vi "Main.vi"(11 "Module Admin":refnum<class "Delacor_lib_QMH_Module Admin.lvclass">) -> ()   [LabVIEW 2020, in "Graficas.lvlib"]
doc: "This template is based off of the Queued Message Handler design pattern and the Queued Message Handler project template that ships with LabVIEW.\n\nThe main difference is that the queue is private to this module and communication between modules is performed via Broadcast and Request events.\n\nRequest events are wrapped in public API methods and are handled in the Event Handling Loop (EHL) of this VI. Any module can register for Broadcast events sent by this module. The EHL generates messages based on user interface actions.\n\nThe Message Handling Loop (MHL) processes messages generated by the EHL, or by other messages. The messages are string values, so new messages can be added easily to the Message Cases case structure in the MHL. Each message cluster can also provide an optional value for Message Data, which is a variant that can be converted to whatever message-specific data is required.\n_____\nBased on Delacor QMH Project Template 5.0.0.82."
uses:
  Graficas.lvlib
  <vilib>/Delacor/Delacor QMH/Libraries/Module Admin_class/Delacor_lib_QMH_Module Admin.lvclass
  Module Data--cluster.ctl
  <vilib>/Delacor/Delacor QMH/Libraries/Message Queue_class/Delacor_lib_QMH_Message Queue.lvclass/Delacor_lib_QMH_Message Queue.ctl
  Stop Argument--cluster.ctl
  <vilib>/Delacor/Delacor QMH/Libraries/Module Admin_class/Delacor_lib_QMH_Module Admin.lvclass/Delacor_lib_QMH_Module Admin.ctl
  Mostrar en SubPanel Argument--cluster.ctl
  <vilib>/Utility/miscctls.llb/LVPointTypeDef.ctl
  <vilib>/Delacor/Delacor QMH/Libraries/Message Queue_class/Delacor_lib_QMH_Enqueue Message (Single).vi
  <vilib>/Delacor/Delacor QMH/Libraries/Module Admin_class/Delacor_lib_QMH_Get External Launch.vi
  <vilib>/Utility/error.llb/Error Cluster From Error Code.vi
  <vilib>/ErrorRing/Error Ring.xnode
  <vilib>/Delacor/Delacor QMH/Libraries/Message Queue_class/Delacor_lib_QMH_Message Queue.lvclass
  Main/Main.lvlib
panel:
  out "Grafica Excitacion":dbl(graph)
  out "Grafica Voltajes":T1(graph)
  out "Grafica SOC":dbl(graph)
  out "Grafica Corriente":dbl(graph)
  out "SOC de Batería":dbl=80.0 format="%_5f %%"
  out "Voltaje de Batería":dbl=270.0 format="%.1f V"
  out "Corriente Excitación":dbl=2.0 format="%_3f A"
  out "Potencia Generador":dbl=300.0 format="%.1f kW"
  out "Corriente Generador":dbl=1000.0 format="%.1f A"
  out "Voltaje Generador":dbl=288.0 format="%.1f V"
  out "error out":errorcluster
  out "Status":string
  # "Tendencias del Generador"
  # "Voltaje Generador / Batería"
  # "Corriente del Generador"
  # "Indicadores Generador"
  # "Estado de Carga de Batería"
  # "Corriente de Excitación"
  # "Indicadores Batería"
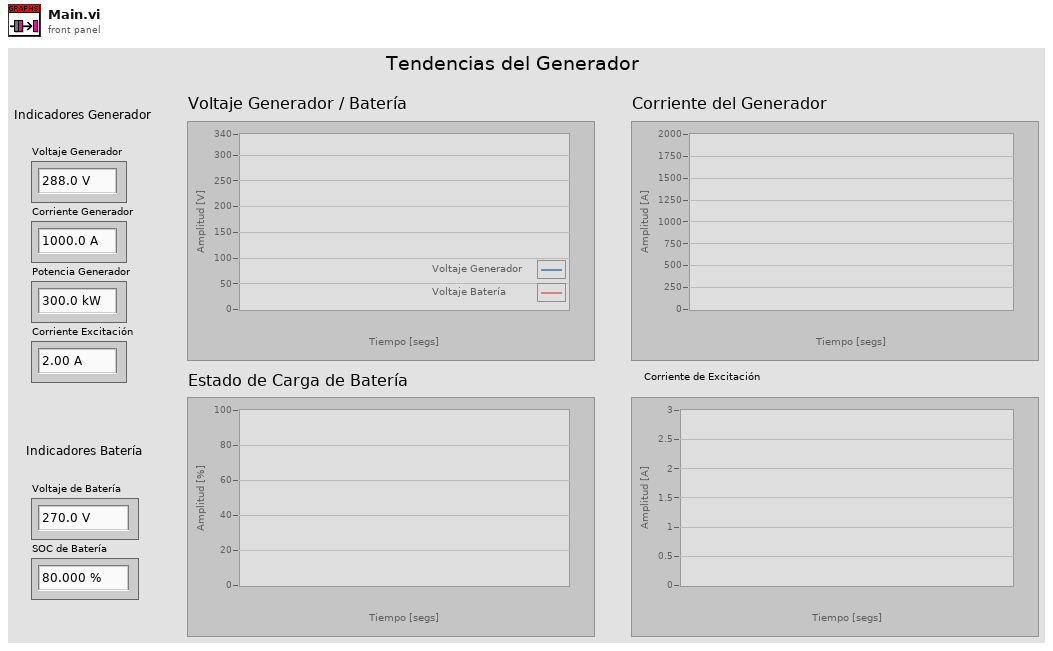
[diagram p1: front panel]
types:
  T1 = cluster{"Voltaje Generador":dbl, "Voltaje de Batería":dbl}
  T2 = typedef "Graficas.lvlib/Request Events--cluster.ctl" = cluster{"Stop Module":refnum<user-event>, "Show Panel":refnum<user-event>, "Hide Panel":refnum<user-event>, "Get Module Execution Status":refnum<user-event>, "Show Diagram":refnum<user-event>, "Mostrar en SubPanel":refnum<user-event>}
  T3 = typedef "Main.lvlib/Broadcast Events--cluster.ctl" = cluster{"Module Did Init":refnum<user-event>, "Status Updated":refnum<user-event>, "Error Reported":refnum<user-event>, "Module Did Stop":refnum<user-event>, "Update Module Execution Status":refnum<user-event>, "Generador Encendido-Apagado":refnum<user-event>}
  T4 = typedef "Graficas.lvlib/Module Data--cluster.ctl" = cluster{"Status":string}
  T5 = enum32{"invalid lock state", "Not Locked", "Locked (No Password)", "Password-protected"}
  T6 = typedef "Graficas.lvlib/Stop Argument--cluster.ctl" = cluster{"Origin":string, "Exit via Stop Module Req?":bool, "Wait for Module to stop?":bool}
  T7 = typedef "Graficas.lvlib/Mostrar en SubPanel Argument--cluster.ctl" = cluster{"SubPnl Refnum":refnum<vi>}
  T8 = cluster{"current time":timestamp, "Voltaje Generador":dbl, dbl}[]
  T9 = typedef "LVPointTypeDef.ctl" = cluster{"Horizontal":i16, "Vertical":i16}
  T10 = enum32{"Invalid", "Standard", "Closed", "Hidden", "Minimized", "Maximized"}
  T11 = cluster{"Voltaje Generador":dbl, "Voltaje de Batería":dbl}[]
  T12 = cluster{"current time":timestamp, "Corriente Generador":dbl}[]
  T13 = enum8{"Enabled", "Disabled", "Disabled and Grayed Out"}
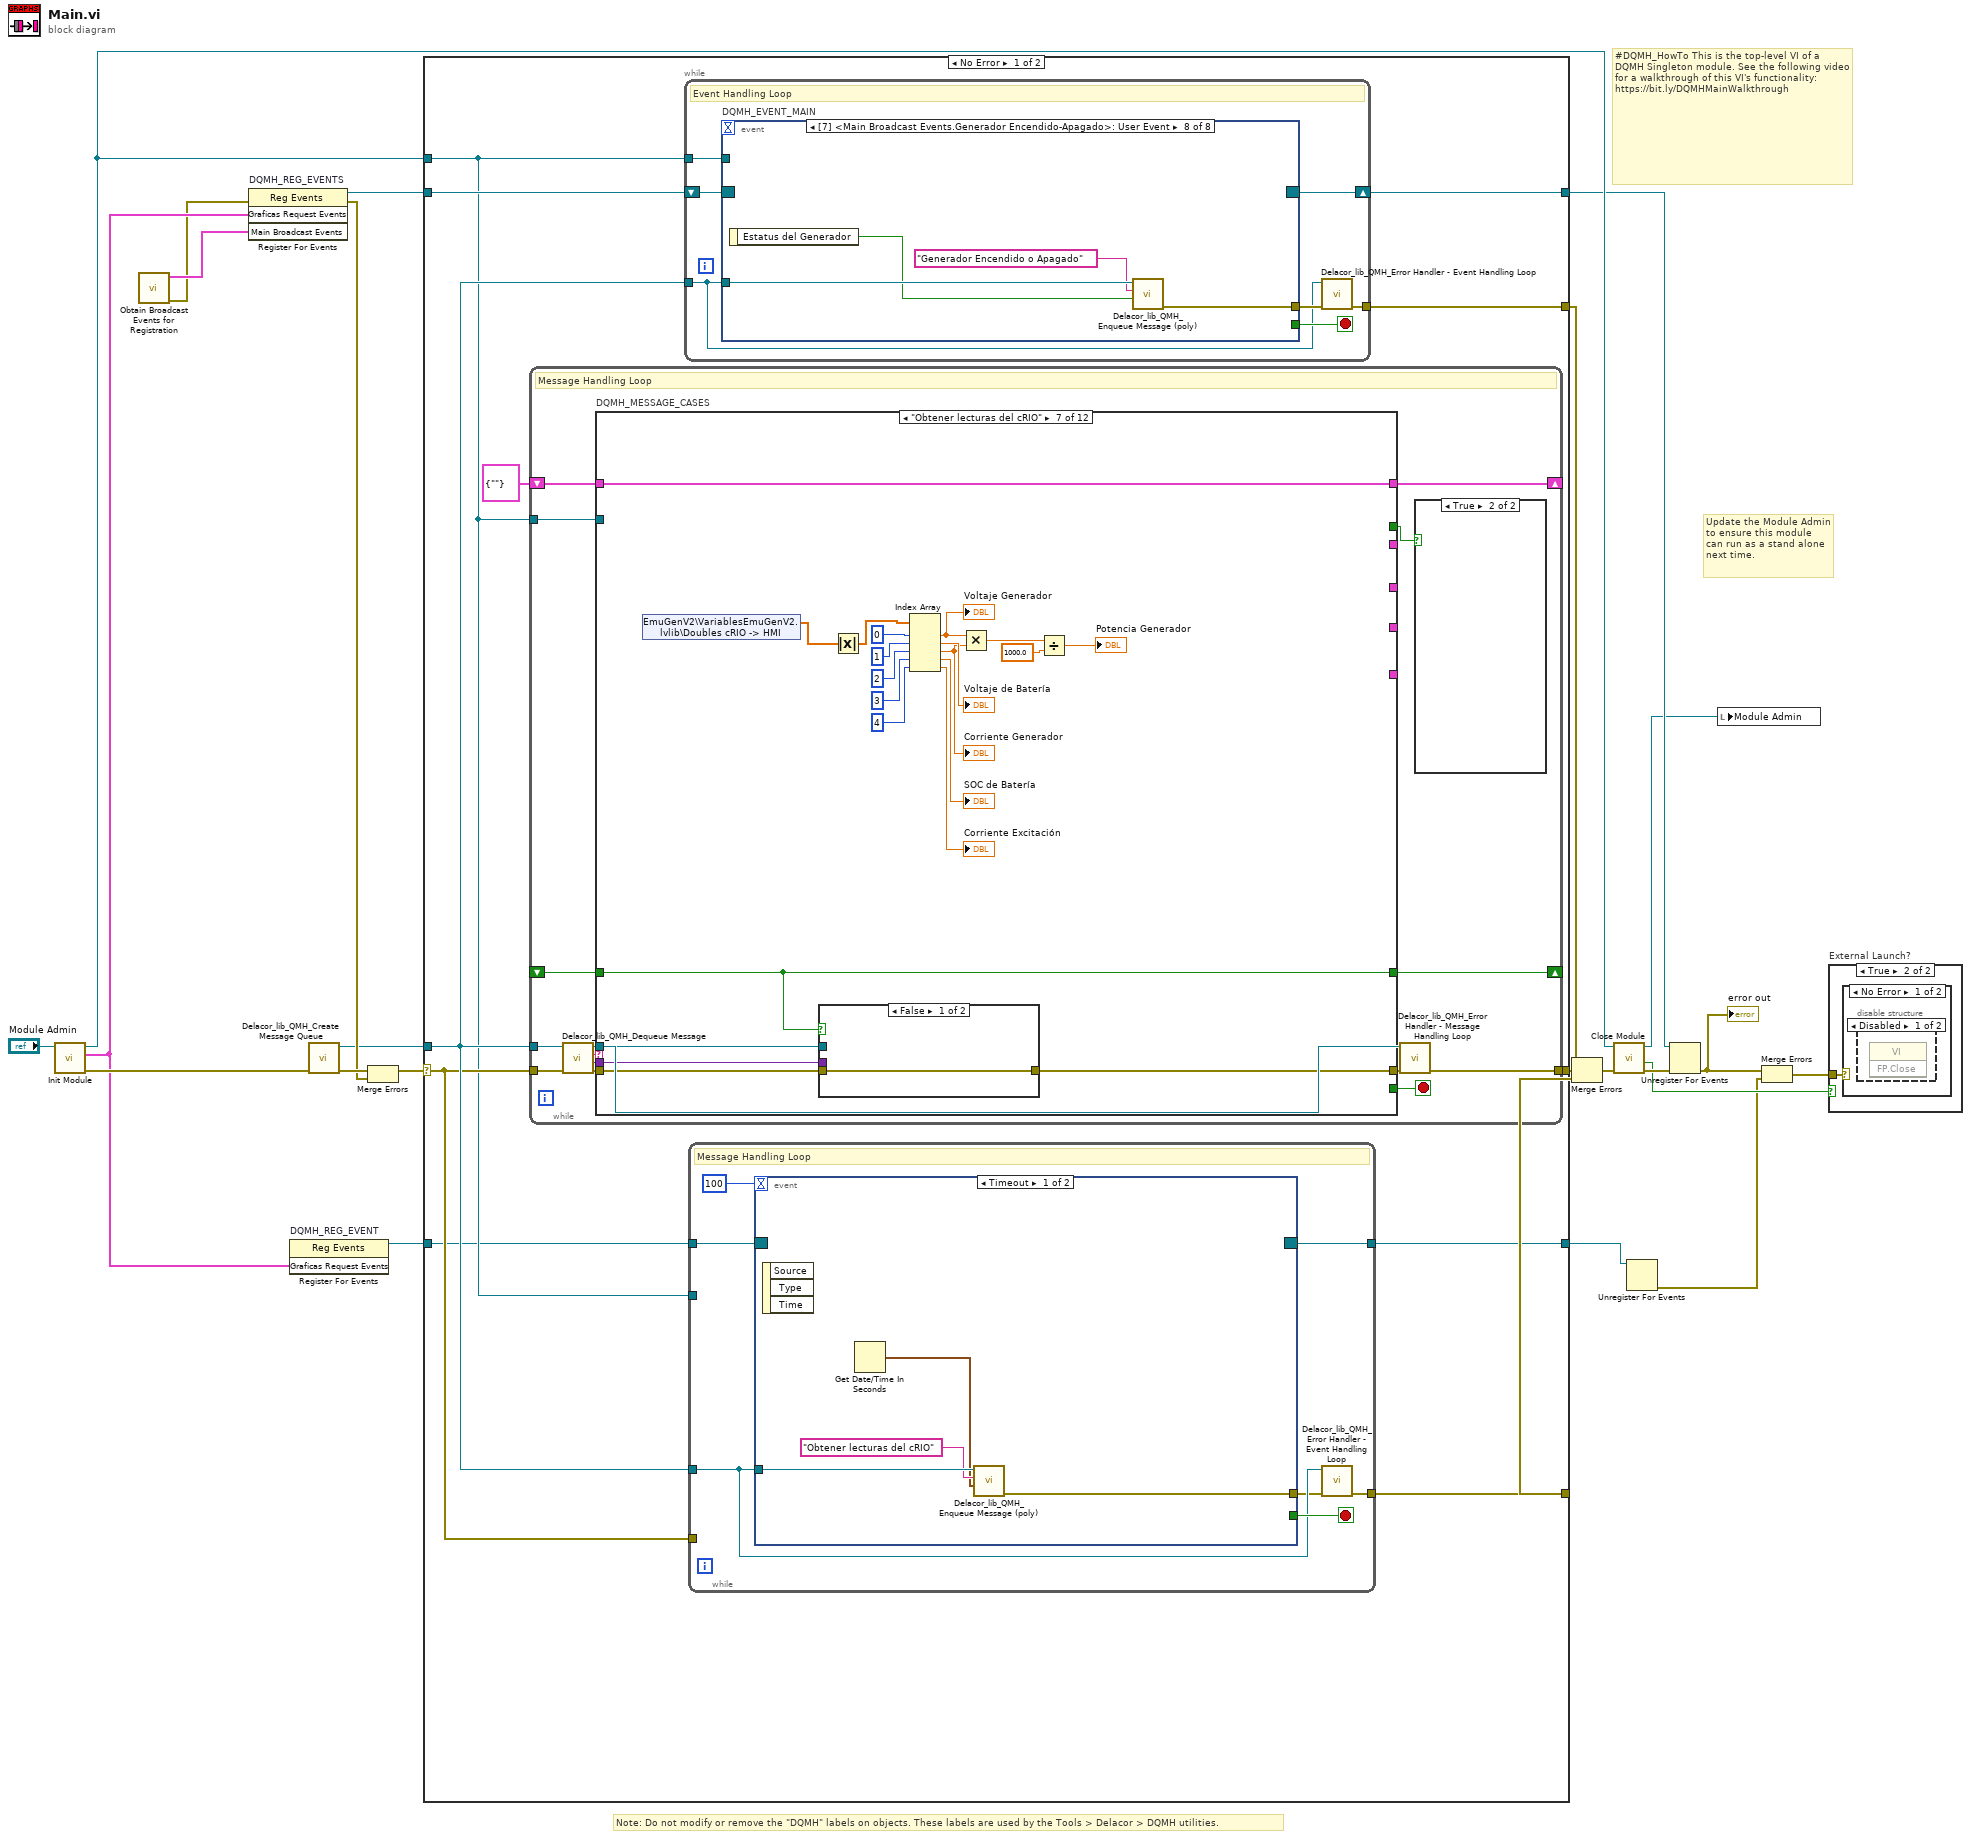
[diagram p0: block diagram]
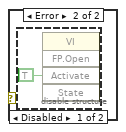
[diagram p4: hidden frame]
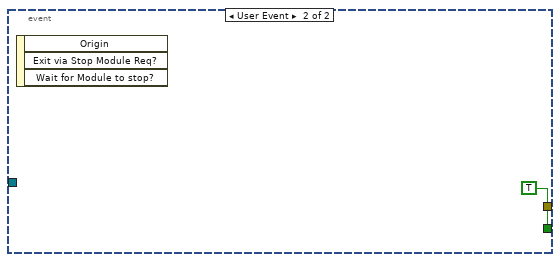
[diagram p6: hidden frame]
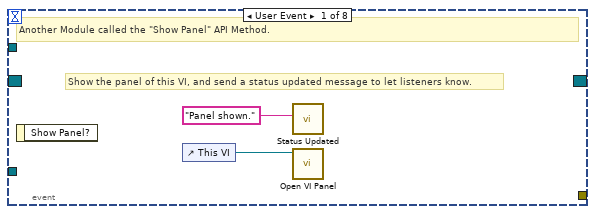
[diagram p7: hidden frame]
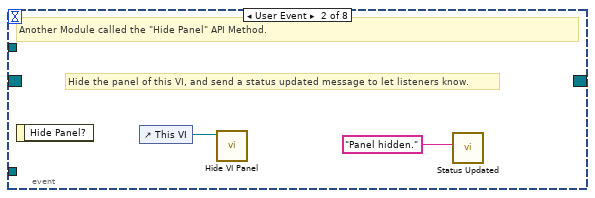
[diagram p8: hidden frame]
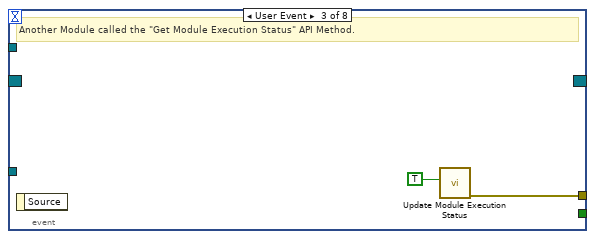
[diagram p9: hidden frame]
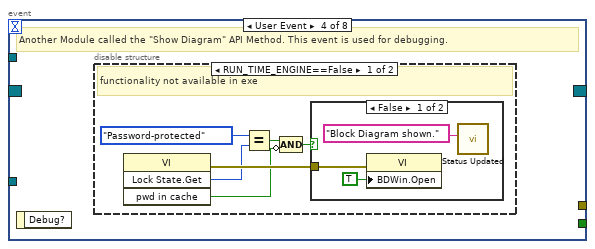
[diagram p10: hidden frame]
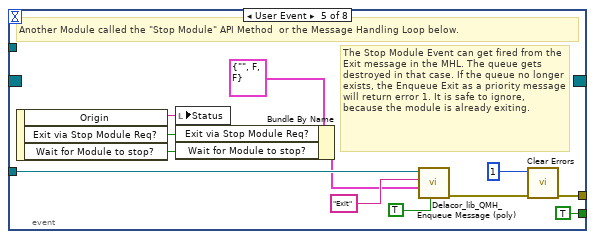
[diagram p13: hidden frame]
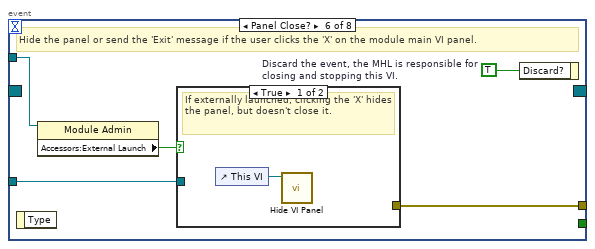
[diagram p14: hidden frame]
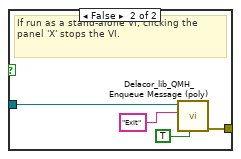
[diagram p15: hidden frame]
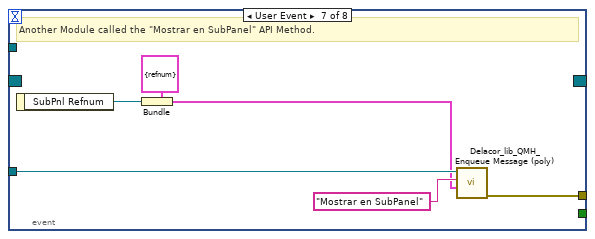
[diagram p16: hidden frame]
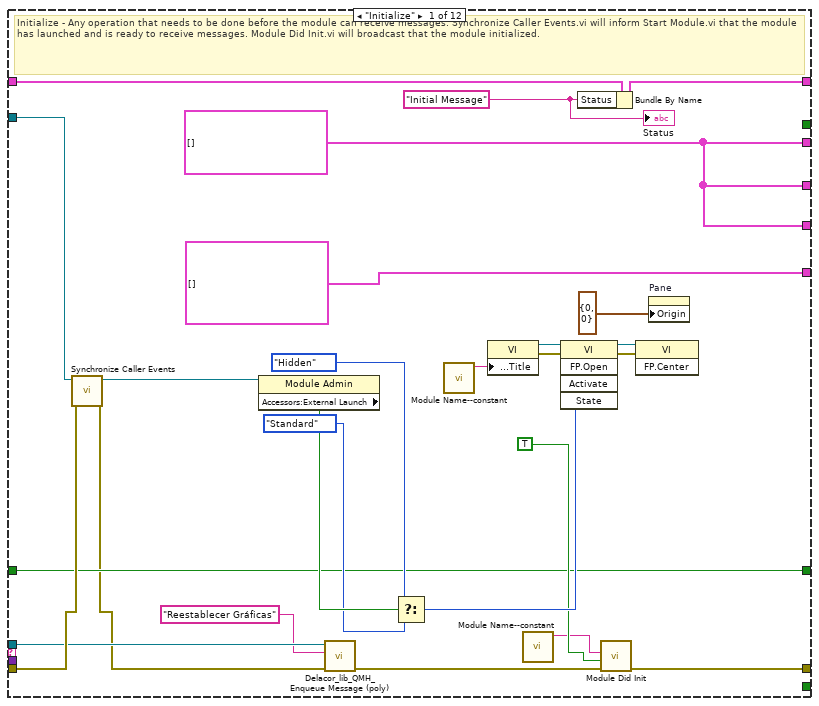
[diagram p18: hidden frame]
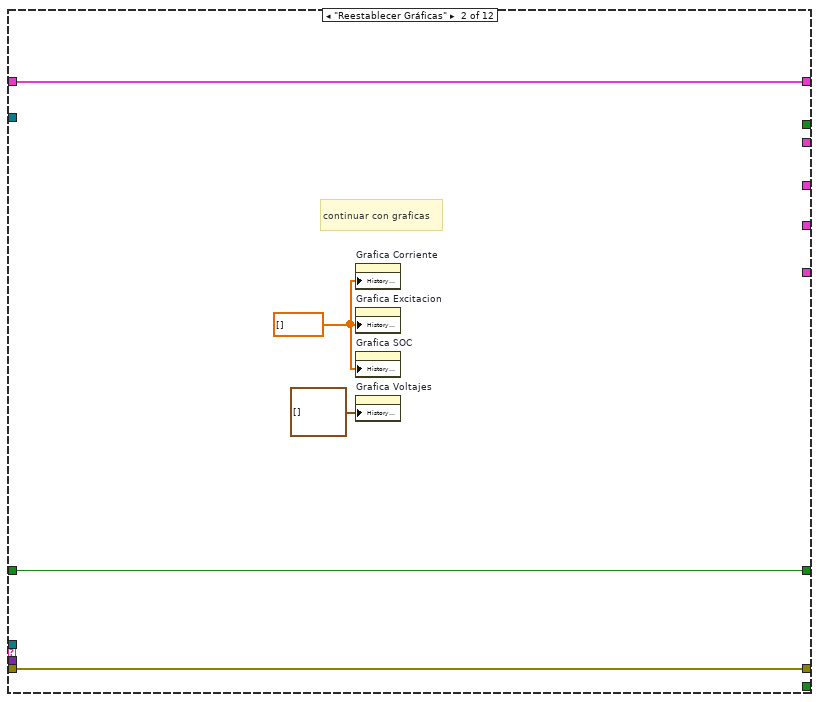
[diagram p19: hidden frame]
diagram:
  # "#DQMH_HowTo This is the top-level VI of a DQMH Singleton module. See the following video for a walkthrough of this VI's functionality: https://bit.ly/DQMHMainWalkthrough"
  # "Note: Do not modify or remove the \"DQMH\" labels on objects. These labels are used by the Tools > Delacor > DQMH utilities."
  # "Update the Module Admin to ensure this module can run as a stand alone next time."
  n1 = call "Init Module.vi"("Singleton Module Admin in"="Module Admin") -> ("error out"=w23:errorcluster, "Graficas Request Events"=w9:T2, "Singleton Module Admin out"=w16:refnum<class "Delacor_lib_QMH_Module Admin.lvclass">)  [unwired: 8 in]
  n2 = call "Obtain Broadcast Events for Registration.vi"() -> ("error out"=w1:errorcluster, "Main Broadcast Events"=w2:T3)  [unwired: 9 in, 1 out]
  n3 = register-events "DQMH_REG_EVENTS"(error in=w1, w9, w2) -> (reference out=w14:refnum<event-registration>, error out=w17:errorcluster)  [unwired: 1 in]
  n4 = register-events "DQMH_REG_EVENT"(w9) -> (reference out=w8:refnum<event-registration>)  [unwired: 2 in, 1 out]
  n5 = call <vilib>:"Delacor_lib_QMH_Create Message Queue.vi"("error in (no error)"=w23) -> ("error out"=w19:errorcluster, "Message Queue"=w13:refnum<class "Delacor_lib_QMH_Message Queue.lvclass">)  [unwired: 9 in]
  n6 = Merge Errors(w19, w17) -> (w18:errorcluster)
  n7 = case shown="No Error" w18 {
    selector: w18 -> [w29 w274]
    tunnel: [w35 w273] -> w24
    tunnel: [w33 w279] -> w15
    tunnel: w14 -> [w31 w279]
    tunnel: w13 -> [w30 w272]
    tunnel: [w34 _] -> w21
    tunnel: w16 -> [w28 w275]
    tunnel: w8 -> [w27 w271]
    tunnel: [w26 w271] -> w7
    tunnel: [w25 _] -> w3
    frame No Error {
      n8 = while {
        tunnel: w30 -> [w107]
        shift-right: [w111] -> _
        shift-left: T4 {"Status"=""} ("Data Cluster") -> [w112]
        tunnel: w29 -> [w115]
        tunnel: [w113] -> w35
        tunnel: w28 -> [w105]
        shift-right: [w103] -> _
        shift-left: _ -> [w102]
        stop <- w110 stop-if-true
        # "Message Handling Loop"
        n9 = call-dynamic "Delacor_lib_QMH_Dequeue Message.vi"("error in (no error)"=w115, "Message Queue in"=w107) -> ("error out"=w114:errorcluster, "Message Data"=w108:variant, "Message"=w109:string, "Message Queue out"=w106:refnum<class "Delacor_lib_QMH_Message Queue.lvclass">)  [unwired: 6 in]
        n10 = case "DQMH_MESSAGE_CASES" shown="\"Obtener lecturas del cRIO\"" w109 {
          selector: w109 -> [_ _ _ _ _ _ _ _ _ _ _ w258]
          tunnel: w106 -> [w120 _ _ _ _ w167 w200 _ _ w226 w249 _]
          tunnel: w114 -> [w140 w147 w150 w160 w164 w171 w199 w218 w221 w233 w255 w260]
          tunnel: [w139 w147 w150 w152 w163 w173 w198 w217 w221 w229 w252 w261] -> w116
          tunnel: w112 -> [w130 w146 w149 w159 w162 w172 w201 w216 w220 w228 w248 w259]
          tunnel: [w129 w146 w149 w159 w162 w172 w201 w216 w220 w228 w248 w259] -> w111
          tunnel: [_ _ _ _ _ _ _ _ _ _ w247 _] -> w110
          tunnel: w108 -> [_ _ _ w158 _ w170 w197 _ _ w227 w246 _]
          tunnel: w105 -> [w131 _ _ _ _ _ _ _ _ w225 w241 _]
          tunnel: [T8 [] _ _ _ _ _ _ _ _ _ _ _] -> _
          tunnel: [w122 _ _ _ _ _ _ _ _ _ _ _] -> _
          tunnel: [w122 _ _ _ _ _ _ _ _ _ _ _] -> _
          tunnel: [w122 _ _ _ _ _ _ _ _ _ _ _] -> _
          tunnel: [_ _ _ _ _ _ _ TRUE _ _ _ _] -> w104
          tunnel: [w121 w145 w148 w151 w161 w165 w196 w214 w219 w222 w240 w256] -> w103
          tunnel: w102 -> [w121 w145 w148 w151 w161 _ w196 w214 w219 w222 w240 w256]
          frame "Initialize" {
            w122 = T12 []
            w124 = "Initial Message" ("Initial Message")
            # "Initialize - Any operation that needs to be done before the module can receive messages. Synchronize Caller Events.vi will inform Start Module.vi that the module has launched and is ready to receive messages. Module Did Init.vi will broadcast that the module initialized."
            n11 = call "Synchronize Caller Events.vi"("error in (no error)"=w140, "Singleton Module Admin in"=w131) -> ("error out"=w119:errorcluster, "Singleton Module Admin out"=w126:refnum<class "Delacor_lib_QMH_Module Admin.lvclass">)  [unwired: 8 in]
            n12 = property class="Module Admin"(reference=w126) -> ("Accessors:External Launch"=w135:bool)  [unwired: 1 in, 2 out]
            n13 = call-poly <vilib>:"Delacor_lib_QMH_Enqueue Message (poly).vi"("error in (no error)"=w119, "Message"="Reestablecer Gráficas", "Message Queue in"=w120) -> ("error out"=w118:errorcluster)  [unwired: 7 in, 1 out]
            n14 = Select(t=T10."Hidden" ("State"), s=w135, f=T10."Standard" ("State")) -> (s? t:f=w132:T10)
            n15 = call "Module Name--constant.vi"() -> ("Module Name"=w138:string)  [unwired: 11 in]
            n16 = property class="VI"("Front Panel.Title"=w138) -> (reference out=w137:refnum<vi>, error out=w142:errorcluster)  [unwired: 2 in]
            n17 = call "Module Name--constant.vi"() -> ("Module Name"=w127:string)  [unwired: 11 in]
            n18 = invoke class="VI" method="FP.Open"(reference=w137, error in=w142, "State"=w132) -> (reference out=w136:refnum<vi>, error out=w141:errorcluster)  [unwired: 2 in, 3 out]
            n19 = Bundle By Name(cluster=w130, "Status"=w124) -> (w129:T4)
            n20 = call "Module Did Init.vi"("error in (no error)"=w118, "Initialized?"=TRUE, "Origin"=w127) -> ("error out"=w139:errorcluster)  [unwired: 8 in]
            n21 = invoke class="VI" method="FP.Center"(reference=w136, error in=w141) -> ()  [unwired: 1 in, 3 out]
            n22 = property on="Pane" class="Pane"("Origin"=T9 {"Horizontal"=0, "Vertical"=0}) -> ()  [unwired: 2 in, 2 out]
            "Status" <- w124
          }
          frame "Reestablecer Gráficas" {
            w144 = dbl[] [] ("History Data")
            # "continuar con graficas"
            n23 = property on="Grafica Corriente" class="WFChart (strict)"("History Data"=w144) -> ()  [unwired: 2 in, 2 out]
            n24 = property on="Grafica Excitacion" class="WFChart (strict)"("History Data"=w144) -> ()  [unwired: 2 in, 2 out]
            n25 = property on="Grafica SOC" class="WFChart (strict)"("History Data"=w144) -> ()  [unwired: 2 in, 2 out]
            n26 = property on="Grafica Voltajes" class="WFChart (strict)"("History Data"=T11 []) -> ()  [unwired: 2 in, 2 out]
          }
          frame "--- Module Specific ---" {
            # "Separator -- The following cases handle messages specific to this Module."
          }
          frame "Mostrar en SubPanel" {
            n27 = Variant To Data(error in=w160, type=T7 {"SubPnl Refnum"=refnum} ("Mostrar en SubPanel Argument"), Variant=w158) -> (data=w156:T7, error out=w153:errorcluster)
            n28 = Unbundle By Name(w156) -> ("SubPnl Refnum"=w155:refnum<vi>)
            n29 = control-ref of="This VI"() -> (w154:refnum<vi>)
            n30 = call "Insert SubPanel.vi"("error in (no error)"=w153, "VI Ref"=w154, "Subpanel Ref"=w155) -> ("error out"=w152:errorcluster)  [unwired: 8 in]
          }
          frame "---Copy This Frame---" {
            # "Duplicate this frame when creating new messages.  Change this comment in the duplicated frame to describe this message."
            n31 = Merge Errors(w164) -> (w163:errorcluster)
          }
          frame "Generador Encendido o Apagado" {
            # "Duplicate this frame when creating new messages.  Change this comment in the duplicated frame to describe this message."
            n32 = Variant To Data(error in=w171, type=FALSE, Variant=w170) -> (data=w165:bool, error out=w169:errorcluster)
            n33 = case shown="False" w165 {
              frame False {
                w179 = T13."Disabled and Grayed Out" ("Disabled")
                n34 = property on="Grafica Corriente" class="WFChart (strict)"("DisabledEnum"=w179) -> ()  [unwired: 2 in, 2 out]
                n35 = property on="Grafica Excitacion" class="WFChart (strict)"("DisabledEnum"=w179) -> ()  [unwired: 2 in, 2 out]
                n36 = property on="Grafica Voltajes" class="WFChart (strict)"("DisabledEnum"=w179) -> ()  [unwired: 2 in, 2 out]
                n37 = property on="Grafica SOC" class="WFChart (strict)"("DisabledEnum"=w179) -> ()  [unwired: 2 in, 2 out]
              }
              frame True {
                w180 = T13."Enabled" ("Disabled")
                n38 = property on="Grafica Corriente" class="WFChart (strict)"("DisabledEnum"=w180) -> ()  [unwired: 2 in, 2 out]
                n39 = property on="Grafica Excitacion" class="WFChart (strict)"("DisabledEnum"=w180) -> ()  [unwired: 2 in, 2 out]
                n40 = property on="Grafica Voltajes" class="WFChart (strict)"("DisabledEnum"=w180) -> ()  [unwired: 2 in, 2 out]
                n41 = property on="Grafica SOC" class="WFChart (strict)"("DisabledEnum"=w180) -> ()  [unwired: 2 in, 2 out]
              }
            }
            n42 = case shown="False" w165 {
              tunnel: w169 -> [w177 w178]
              tunnel: [w176 w178] -> w168
              tunnel: w167 -> [w174 _]
              frame False {
                n43 = call-poly <vilib>:"Delacor_lib_QMH_Enqueue Message (poly).vi"("error in (no error)"=w177, "Message"="Reestablecer Gráficas", "Message Queue in"=w174) -> ("error out"=w176:errorcluster)  [unwired: 7 in, 1 out]
              }
              frame True {
              }
            }
            n44 = Merge Errors(w168) -> (w173:errorcluster)
          }
          frame "Obtener lecturas del cRIO" {
            n45 = shared-variable "EmuGenV2\\VariablesEmuGenV2.lvlib\\Doubles cRIO -> HMI"() -> (w182:dbl[])  [unwired: 1 in, 1 out]
            n46 = case shown="False" w196 {
              tunnel: w200 -> [_ w207]
              tunnel: w199 -> [w202 w205]
              tunnel: [w202 w204] -> w198
              tunnel: w197 -> [_ w203]
              frame False {
              }
              frame True {
                n47 = call-poly <vilib>:"Delacor_lib_QMH_Enqueue Message (poly).vi"("error in (no error)"=w205, "Message Data"=w203, "Message"="Actualizar Graficas", "Message Queue in"=w207) -> ("error out"=w204:errorcluster)  [unwired: 6 in, 1 out]
              }
            }
            n48 = Absolute Value(x=w182) -> (abs(x)=w181:dbl[])
            n49 = Index Array(array=w181, index #1=0 ("index"), index #2=1 ("index"), index #3=2 ("index"), index #4=3 ("index"), index #5=4 ("index")) -> (element #1=w188:dbl, element #2=→"Voltaje de Batería":dbl, element #3=w186:dbl, element #4=→"SOC de Batería":dbl, element #5=→"Corriente Excitación":dbl)
            "Voltaje Generador" <- w188
            "Corriente Generador" <- w186
            n50 = Multiply(x=w188, y=w186) -> (x*y=w185:dbl)
            n51 = Divide(x=w185, y=1000.0) -> (x/y=→"Potencia Generador":dbl)
          }
          frame "Actualizar Graficas" {
            # "Duplicate this frame when creating new messages.  Change this comment in the duplicated frame to describe this message."
            n52 = local read "Voltaje Generador"() -> (w212:dbl)
            n53 = local read "Voltaje de Batería"() -> (w209:dbl)
            n54 = local read "SOC de Batería"() -> (→"Grafica SOC":dbl)
            n55 = local read "Corriente Generador"() -> (→"Grafica Corriente":dbl)
            n56 = local read "Corriente Excitación"() -> (→"Grafica Excitacion":dbl)
            n57 = Bundle("Voltaje Generador"=w212, "Voltaje de Batería"=w209) -> (→"Grafica Voltajes":T1)  [unwired: 1 in]
            n58 = Merge Errors(w218) -> (w217:errorcluster)
          }
          frame "--- Exit and Error Handling---" {
            # "Separator - The following cases handle errors and exit messages."
          }
          frame "Error" {
            # "#CodeRecommended - If you ever change the name of this \"Error\" message, you'll need to update the name in the Check Loop Error.vi as well."
            # "#CodeRecommended - If the module is running in standalone mode (External Launch = FALSE), this code will pop up an error dialog and call the 'Exit' message if an error occurs. Add more fine-grained error handling here."
            # "Error - Check the error message data and respond accordingly. This message is sent by the \"Error Handler\" VIs at the end of each loop in this application."
            n59 = property class="Module Admin"(reference=w225) -> ("Accessors:External Launch"=w224:bool)  [unwired: 1 in, 2 out]
            n60 = Variant To Data(error in=w233, type=errorcluster {"status"=FALSE, "code"=0, "source"=""} ("error constant"), Variant=w227) -> (data=w234:errorcluster, error out=w231:errorcluster)
            n61 = call "Module Name--constant.vi"() -> ("Module Name"=w223:string)  [unwired: 11 in]
            n62 = call "Error Reported.vi"("Additional Information"=w223, "Error"=w234) -> ()  [unwired: 9 in, 1 out]
            n63 = case shown="False" w224 {
              tunnel: [w239 _] -> w230
              tunnel: w226 -> [w237 _]
              tunnel: w234 -> [w238 _]
              frame False {
                # "If the module is running standalone, then pop up an error dialog and call the \"Exit\" message."
                n64 = call <vilib>:"Simple Error Handler.vi"("error in (no error)"=w238) -> ()  [unwired: 4 in, 5 out]
                n65 = call-poly <vilib>:"Delacor_lib_QMH_Enqueue Message (poly).vi"("Priority Message? (F)"=TRUE, "Message"="Exit", "Message Queue in"=w237) -> ("error out"=w239:errorcluster)  [unwired: 7 in, 1 out]
              }
              frame True {
                # "If the module was launched externally, calling the Error Reported broadcast VI is the only action performed by the \"Error\" message. The module's caller can then process the error appropriately."
              }
            }
            n66 = Merge Errors(w231, w230) -> (w229:errorcluster)
            n67 = local write "error out"(w229) -> ()
          }
          frame "Exit" {
            w245 = 91  # 91: not all Exit messages will have an argument
            w247 = TRUE  # Stop the VI
            # "Release the message queue reference"
            # "#CodeNeeded - Add any required cleanup code here"
            # "Exit - Exit the application."
            n68 = Variant To Data(error in=w255, type=T6 {"Origin"="", "Exit via Stop Module Req?"=FALSE, "Wait for Module to stop?"=FALSE} ("Stop Argument"), Variant=w246) -> (data=w243:T6, error out=w251:errorcluster)
            n69 = call <vilib>:"Clear Errors.vi"("error in (no error)"=w251, "specific error code to clear (0: all)"=w245) -> ("error out"=w254:errorcluster)  [unwired: 4 in, 1 out]
            n70 = control-ref of="This VI"() -> (w242:refnum<vi>)
            n71 = call-dynamic "Delacor_lib_QMH_Release Message Queue.vi"("error in (no error)"=w254, "Message Queue"=w249) -> ("error out"=w253:errorcluster)  [unwired: 9 in]
            n72 = call "Handle Exit.vi"("Stop Argument"=w243, "Admin in"=w241, "VI reference"=w242) -> ("error out"=w250:errorcluster)  [unwired: 7 in, 1 out]
            n73 = Merge Errors(w253, w250) -> (w252:errorcluster)
          }
          frame Default {
            # "'Default' case only runs if there is a message that isn't defined in any of the other cases.  Output a programming error."
            n74 = call "Module Name--constant.vi"() -> ("Module Name"=w257:string)  [unwired: 11 in]
            n75 = xnode "Error Ring"("parameter 0"=w258, "parameter 1"=w257) -> ("error out"=w262:errorcluster)
            n76 = Merge Errors(w260, w262) -> (w261:errorcluster)
          }
        }
        n77 = call-dynamic "Delacor_lib_QMH_Error Handler - Message Handling Loop.vi"("error in (no error)"=w116, "Message Queue in"=w106) -> ("dup error in"=w113:errorcluster)  [unwired: 8 in, 1 out]
        n78 = case shown="True" w104 {
          frame False {
          }
          frame True {
          }
        }
      }
      n79 = while {
        tunnel: w30 -> [w48]
        shift-right: [w51] -> w33
        shift-left: w31 -> [w52]
        tunnel: [w53] -> w34
        tunnel: w28 -> [w49]
        stop <- w50 stop-if-true
        # "Event Handling Loop"
        n80 = event "DQMH_EVENT_MAIN" shown="[7] <Main Broadcast Events.Generador Encendido-Apagado>: User Event" {
          selector: w52 -> [_ _ _ _ _ _ _ _]
          dyn-events: [_ _ _ _ _ _ _ _] -> w51
          timeout: _ -> [_ _ _ _ _ _ _ _]
          tunnel: [_ _ _ _ TRUE ("Discard?") _ _ _] -> w50
          tunnel: w48 -> [_ _ _ _ w77 w84 w97 w101]
          tunnel: [_ _ w60 _ w80 w86 w92 w100] -> w54
          tunnel: w49 -> [_ _ _ _ _ w83 _ _]
          event User Event {
            # "Show the panel of this VI, and send a status updated message to let listeners know."
            # "Another Module called the \"Show Panel\" API Method."
            n81 = event-data() -> ()  [unwired: 1 in, 1 out]
            n82 = control-ref of="This VI"() -> (w56:refnum<vi>)
            n83 = call "Status Updated.vi"("Status"="Panel shown." ("format string")) -> ()  [unwired: 10 in, 1 out]
            n84 = call "Open VI Panel.vi"("VI"=w56) -> ()  [unwired: 10 in, 1 out]
          }
          event User Event {
            # "Hide the panel of this VI, and send a status updated message to let listeners know."
            # "Another Module called the \"Hide Panel\" API Method."
            n85 = event-data() -> ()  [unwired: 1 in, 1 out]
            n86 = control-ref of="This VI"() -> (w58:refnum<vi>)
            n87 = call "Hide VI Panel.vi"("VI"=w58) -> ()  [unwired: 10 in, 1 out]
            n88 = call "Status Updated.vi"("Status"="Panel hidden." ("format string")) -> ()  [unwired: 10 in, 1 out]
          }
          event User Event {
            # "Another Module called the \"Get Module Execution Status\" API Method."
            n89 = event-data() -> ()  [unwired: 1 in, 1 out]
            n90 = call "Update Module Execution Status.vi"("Running?"=TRUE) -> ("error out"=w60:errorcluster)  [unwired: 10 in]
          }
          event User Event {
            # "Another Module called the \"Show Diagram\" API Method. This event is used for debugging."
            n91 = event-data() -> ()  [unwired: 1 in, 1 out]
            n92 = disable-structure shown="RUN_TIME_ENGINE==False" {
              frame condition #0 (active) {
                # "functionality not available in exe"
                n93 = invoke class="VI" method="Lock State.Get"() -> (error out=w66:errorcluster, "Get Lock State"=w65:T5, "pwd in cache"=w62:bool)  [unwired: 4 in, 1 out]
                n94 = Equal?(x=T5."Password-protected", y=w65) -> (x = y?=w63:bool)
                n95 = Compound Arithmetic op=AND(w63, invert w62) -> (w61:bool)
                n96 = case shown="False" w61 {
                  tunnel: w66 -> [w69 _]
                  frame False {
                    n97 = property class="VI"(error in=w69, "BDWin.Open"=TRUE ("Block Diagram Window:Open")) -> ()  [unwired: 1 in, 2 out]
                    n98 = call "Status Updated.vi"("Status"="Block Diagram shown." ("format string")) -> ()  [unwired: 10 in, 1 out]
                  }
                  frame True {
                    # "Password-protected VI, and the password is not in the cache. Do not show the diagram."
                  }
                }
              }
              frame condition #1 {
              }
            }
          }
          event User Event {
            # "The Stop Module Event can get fired from the Exit message in the MHL. The queue gets destroyed in that case. If the queue no longer exists, the Enqueue Exit as a priority message will return error 1. It is safe to ignore, because the module is already exiting."
            # "Another Module called the \"Stop Module\" API Method  or the Message Handling Loop below."
            n99 = event-data() -> ("Origin"=w76:string, "Exit via Stop Module Req?"=w72:bool, "Wait for Module to stop?"=w71:bool)  [unwired: 1 in]
            n100 = local write "Status"(w76) -> ()
            n101 = Bundle By Name(cluster=T6 {"Origin"="", "Exit via Stop Module Req?"=FALSE, "Wait for Module to stop?"=FALSE} ("Stop Argument"), "Exit via Stop Module Req?"=w72, "Wait for Module to stop?"=w71) -> (w70:T6)
            n102 = call-poly <vilib>:"Delacor_lib_QMH_Enqueue Message (poly).vi"("Priority Message? (F)"=TRUE, "Message Data"=w70, "Message"="Exit", "Message Queue in"=w77) -> ("error out"=w81:errorcluster)  [unwired: 6 in, 1 out]
            n103 = call <vilib>:"Clear Errors.vi"("error in (no error)"=w81, "specific error code to clear (0: all)"=1) -> ("error out"=w80:errorcluster)  [unwired: 4 in, 1 out]
          }
          event Panel Close? {
            w85 = TRUE  # Discard the event, the MHL is responsible for closing and stopping this VI.
            # "Hide the panel or send the 'Exit' message if the user clicks the 'X' on the module main VI panel."
            n104 = event-data() -> ()  [unwired: 1 in, 1 out]
            n105 = property class="Module Admin"(reference=w83) -> ("Accessors:External Launch"=w82:bool)  [unwired: 1 in, 2 out]
            n106 = case shown="True" w82 {
              tunnel: w84 -> [_ w90]
              tunnel: [_ w91] -> w86
              frame True {
                # "If externally launched, clicking the 'X' hides the panel, but doesn't close it."
                n107 = control-ref of="This VI"() -> (w87:refnum<vi>)
                n108 = call "Hide VI Panel.vi"("VI"=w87) -> ()  [unwired: 10 in, 1 out]
              }
              frame False {
                # "If run as a stand-alone VI, clicking the panel 'X' stops the VI."
                n109 = call-poly <vilib>:"Delacor_lib_QMH_Enqueue Message (poly).vi"("Priority Message? (F)"=TRUE, "Message"="Exit", "Message Queue in"=w90) -> ("error out"=w91:errorcluster)  [unwired: 7 in, 1 out]
              }
            }
            n110 = event-data("Discard?"=w85) -> ()  [unwired: 1 in, 1 out]
          }
          event User Event {
            # "Another Module called the \"Mostrar en SubPanel\" API Method."
            n111 = event-data() -> ("SubPnl Refnum"=w93:refnum<vi>)  [unwired: 1 in]
            n112 = Bundle(cluster=T7 {"SubPnl Refnum"=refnum} ("Mostrar en SubPanel Argument"), "SubPnl Refnum"=w93) -> (w94:T7)
            n113 = call-poly <vilib>:"Delacor_lib_QMH_Enqueue Message (poly).vi"("Message Data"=w94, "Message"="Mostrar en SubPanel", "Message Queue in"=w97) -> ("error out"=w92:errorcluster)  [unwired: 7 in, 1 out]
          }
          event User Event {
            n114 = event-data() -> ("Estatus del Generador"=w99:bool)  [unwired: 1 in]
            n115 = call-poly <vilib>:"Delacor_lib_QMH_Enqueue Message (poly).vi"("Message Data"=w99, "Message"="Generador Encendido o Apagado", "Message Queue in"=w101) -> ("error out"=w100:errorcluster)  [unwired: 7 in, 1 out]
          }
        }
        n116 = call-dynamic "Delacor_lib_QMH_Error Handler - Event Handling Loop.vi"("error in (no error)"=w54, "Message Queue in"=w48) -> ("dup error in"=w53:errorcluster)  [unwired: 8 in, 1 out]
      }
      n117 = while {
        tunnel: w30 -> [w38]
        tunnel: w29 -> [_]
        tunnel: w28 -> [_]
        tunnel: w27 -> [w41]
        tunnel: [w40] -> w26
        tunnel: [w36] -> w25
        stop <- w39 stop-if-true
        # "Message Handling Loop"
        n118 = event shown="[0] Timeout" {
          selector: w41 -> [_ _]
          dyn-events: [_ _] -> w40
          timeout: 100 -> [_ _]
          tunnel: [_ TRUE] -> w39
          tunnel: w38 -> [w46 _]
          tunnel: [w44 _] -> w37
          event Timeout {
            n119 = event-data() -> ()  [unwired: 1 in, 3 out]
            n120 = Get Date/Time In Seconds() -> (seconds since 1Jan1904=w43:timestamp)
            n121 = call-poly <vilib>:"Delacor_lib_QMH_Enqueue Message (poly).vi"("Message Data"=w43, "Message"="Obtener lecturas del cRIO", "Message Queue in"=w46) -> ("error out"=w44:errorcluster)  [unwired: 7 in, 1 out]
          }
          event User Event {
            n122 = event-data() -> ()  [unwired: 1 in, 3 out]
          }
        }
        n123 = call-dynamic "Delacor_lib_QMH_Error Handler - Event Handling Loop.vi"("error in (no error)"=w37, "Message Queue in"=w38) -> ("dup error in"=w36:errorcluster)  [unwired: 8 in, 1 out]
      }
    }
    frame Error {
      # "Synchronize Caller Events.vi will inform Start Module.vi that the module has launched and will let the code calling Start Module.vi register for broadcasts and would permit the caller receive the broadcast that an error occurred at launch time."
      n124 = call-dynamic "Delacor_lib_QMH_Release Message Queue.vi"("error in (no error)"=w274, "Message Queue"=w272) -> ("error out"=w273:errorcluster)  [unwired: 9 in]
      n125 = call "Synchronize Caller Events.vi"("Singleton Module Admin in"=w275) -> ("error out"=w280:errorcluster)  [unwired: 9 in, 1 out]
      n126 = call "Module Name--constant.vi"() -> ("Module Name"=w278:string)  [unwired: 11 in]
      n127 = Format Into String(format string="An error occurred during initialization. %s is no longer running.", w278) -> (resulting string=w276:string)  [unwired: 2 in, 1 out]
      n128 = Merge Errors(w273, w280) -> (w281:errorcluster)
      n129 = call "Error Reported.vi"("Additional Information"=w276, "Error"=w281) -> ()  [unwired: 9 in, 1 out]
    }
  }
  n130 = Merge Errors(w21, w24, w3) -> (w20:errorcluster)
  n131 = call "Close Module.vi"("error in (no error)"=w20, "Module Admin in"=w16) -> ("error out"=w22:errorcluster, "External Launch"=w10:bool, "Module Admin out"=w11:refnum<class "Delacor_lib_QMH_Module Admin.lvclass">)  [unwired: 7 in]
  n132 = Unregister For Events(event registration refnum=w7) -> (error out=w5:errorcluster)  [unwired: 1 in]
  n133 = Unregister For Events(event registration refnum=w15, error in=w22) -> (error out=w6:errorcluster)
  "error out" <- w6
  n134 = local write "Module Admin"(w11) -> ()
  n135 = Merge Errors(w6, w5) -> (w4:errorcluster)
  n136 = case "External Launch?" shown="True" w10 {
    tunnel: w4 -> [_ w282]
    frame False {
    }
    frame True {
      n137 = case shown="No Error" w282 {
        frame No Error {
          n138 = disable-structure shown="Disabled" {
            frame Disabled {
              n139 = invoke class="VI" method="FP.Close"() -> ()  [unwired: 3 in, 3 out]
            }
            frame Enabled {
            }
          }
        }
        frame Error {
          n140 = disable-structure shown="Disabled" {
            frame Disabled {
              n141 = invoke class="VI" method="FP.Open"("Activate"=TRUE ("Activate?")) -> ()  [unwired: 4 in, 5 out]
            }
            frame Enabled {
            }
          }
        }
      }
    }
  }
